vi "Setup.vi"(8 "error in (no error)":errorcluster, 11 "Test Case In":refnum<class "Hungry Hippo Test.lvclass">) -> (0 "error out":errorcluster, 3 "Test Case Out":refnum<class "Hungry Hippo Test.lvclass">)   [LabVIEW 2020, in "Hungry Hippo Test.lvclass"]
uses:
  Hungry Hippo Test.lvclass
  C:/Users/anton/Documents/GitHub/LUnit/source/Examples/Test Inheritance/Animal Test Classes/Animal Test/Animal Test.lvclass
  Animal Classes/Hungry Hippo/Hungry Hippo.lvclass
  C:/Users/anton/Documents/GitHub/LUnit/source/Examples/Test Inheritance/Animal Classes/Animal/Animal.lvclass
  Animal Test/Animal Test.lvclass/Animal Test.ctl
  Animal Test/Animal Test.lvclass
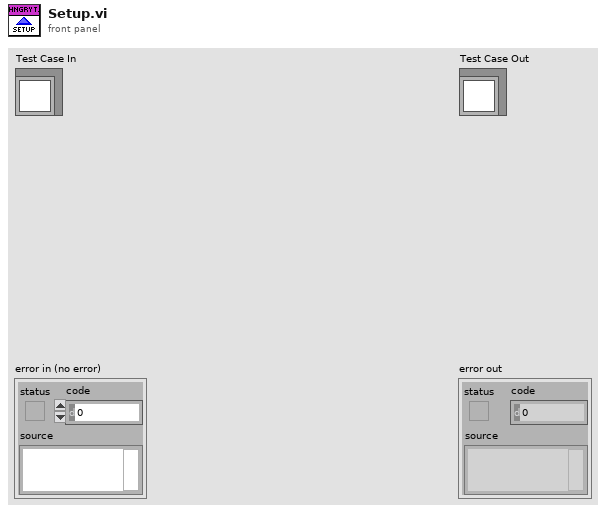
[diagram p1: front panel]
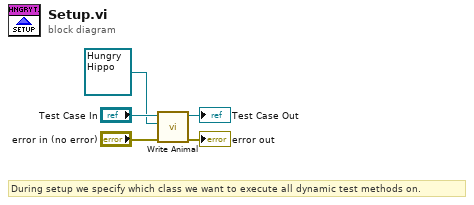
[diagram p0: block diagram]
diagram:
  # "During setup we specify which class we want to execute all dynamic test methods on."
  n1 = call "Write Animal.vi"("error in (no error)"="error in (no error)", "Animal.lvclass"=refnum<class "Hungry Hippo.lvclass"> refnum ("Hungry Hippo.lvclass"), "Animal Test In"="Test Case In") -> ("error out"=→"error out":errorcluster, "Animal Test Out"=→"Test Case Out":refnum<class "Hungry Hippo Test.lvclass">)  [unwired: 7 in]
